vi "Dispose.vi"(8 "Error In":errorcluster, 11 "reference in":refnum<class "Clippy.lvclass">) -> (0 "Error Out":errorcluster, 3 "reference out":refnum<class "Clippy.lvclass">)   [LabVIEW 2020, in "Clippy.lvclass"]
uses:
  Clippy.lvclass
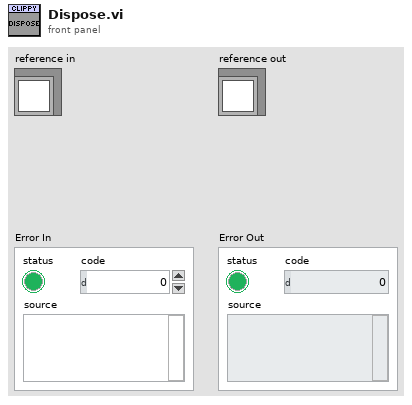
[diagram p1: front panel]
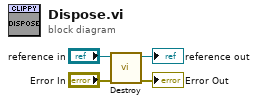
[diagram p0: block diagram]
diagram:
  n1 = call-dynamic "Destroy.vi"("error in (no error)"="Error In", "reference in"="reference in") -> ("error out"=→"Error Out":errorcluster, "reference out"=→"reference out":refnum<class "Clippy.lvclass">)  [unwired: 8 in]
